vi "Normal Example Template.vi"() -> (3 "ImgOut":T1(plugin-control))   [LabVIEW 2014]
doc: "Use this template to build a VI to use as a subVI."
panel:
  # ":: MVi Framework V1.0 ::\nAuthor:Gaoke Yang\nEmail: gaoke.yang@yahoo.com\nWeb: www.mvicontrol.com\nCopyright (C) 2015, MVI Technologies All Rights Reserved"
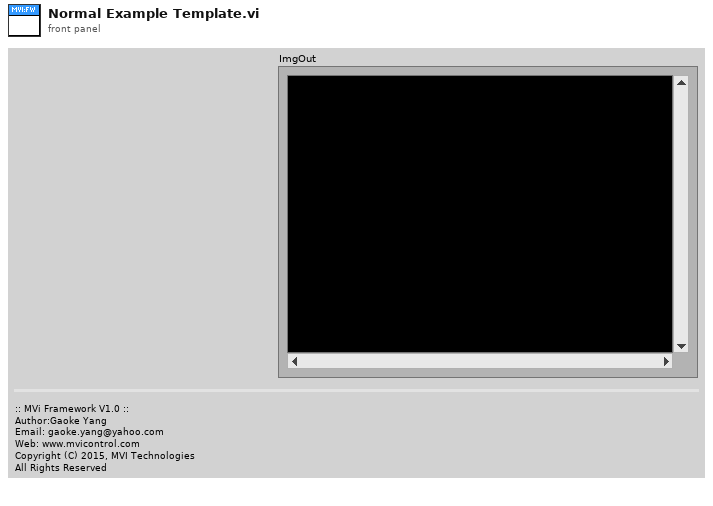
[diagram p1: front panel]
types:
  T1 = typedef "IMAQ Image.ctl" = refnum<image>
  T2 = typedef "Image Type" = u32
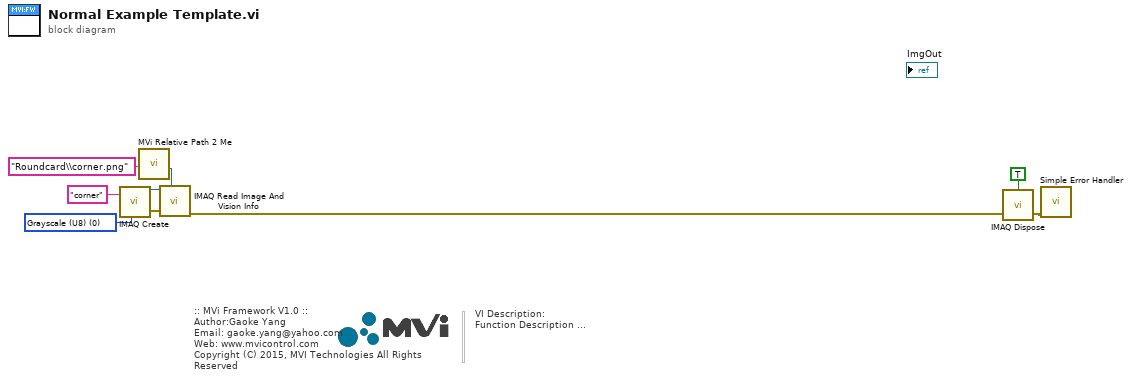
[diagram p0: block diagram]
diagram:
  w9 = T2 0 items=["Grayscale (U8)", "Grayscale (I16)", "Grayscale (SGL)", "Complex (CSG)", "RGB (U32)", "HSL (U32)", "RGB (U64)", "Grayscale (U16)"] ("Image Type")
  # "VI Description:\nFunction Description ..."
  # ":: MVi Framework V1.0 ::\nAuthor:Gaoke Yang\nEmail: gaoke.yang@yahoo.com\nWeb: www.mvicontrol.com\nCopyright (C) 2015, MVI Technologies All Rights Reserved"
  n1 = call "IMAQ Create"("Image Name"="corner" ("name or relative path"), "Image Type"=w9) -> ("New Image"=w8:T1, "error out"=w7:errorcluster)  [unwired: 2 in, 1 out]
  n2 = call "MVi Relative Path 2 Me.vi"("Relative Path"="Roundcard\\corner.png" ("name or relative path")) -> ("Appended Dir"=w5:path)  [unwired: 5 in, 1 out]
  n3 = call "IMAQ Read Image And Vision Info"("File Path"=w5, "error in (no error)"=w7, "Image"=w8) -> ("error out"=w1:errorcluster)  [unwired: 1 in, 7 out]
  n4 = call "IMAQ Dispose"("All Images? (No)"=TRUE, "error in (no error)"=w1) -> ("error out"=w2:errorcluster)  [unwired: 1 in, 3 out]
  n5 = call <vilib>:"Simple Error Handler.vi"("error in (no error)"=w2) -> ()  [unwired: 1 in, 8 out]
